vi "Get Tube Position Arrays.vi"(10 "PPR":i32=1024, 11 "Position Array":T2[](array[typedef])=[{"Positions"=enum."Tube Red A", "Count"=47}, {"Positions"=enum."Tube Black F", "Count"=213}, {"Positions"=enum."Tube Red E", "Count"=383}, {"Positions"=enum."Tube Black D", "Count"=557}, {"Positions"=enum."Tube Red C", "Count"=724}, {"Positions"=enum."Tube Black B", "Count"=898}]) -> (2 "Counts":i32[](array[numeric]), 3 "Positons":T1[](array[typedef]))   [LabVIEW 2020, in "Tube Wheel_ACT.lvlib"]
uses:
  Tube Wheel_ACT.lvlib
  Type Defs/Cluster_Tube Wheel Positions.ctl
  Shared Code/TypeDefs/ENUM_Tube Wheel Positions.ctl
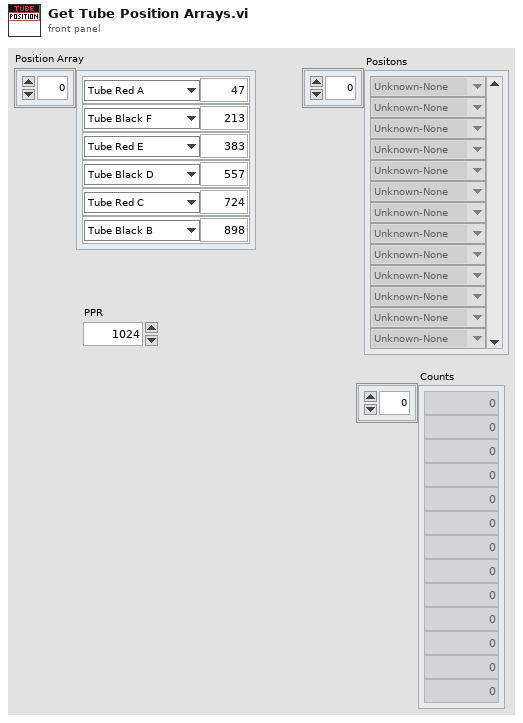
[diagram p1: front panel]
types:
  T1 = typedef "ENUM_Tube Wheel Positions.ctl" = enum16{"Unknown-None", "Tube Red A", "Tube Black B", "Tube Red C", "Tube Black D", "Tube Red E", "Tube Black F", "Load A-B", "Load B-C", "Load C-D", "Load D-E", "Load E-F", "Load F-A"}
  T2 = typedef "Cluster_Tube Wheel Positions.ctl" = cluster{"Positions":T1, "Count":i32}
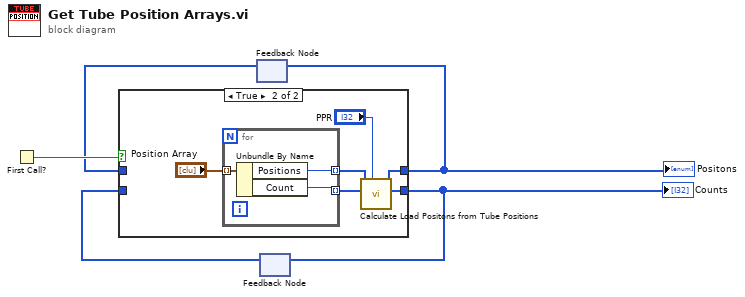
[diagram p0: block diagram]
diagram:
  n1 = First Call?() -> (First Call?: T/F=w5:bool)
  n2 = feedback #1() -> (w2:T1[])  [unwired: 1 in]
  n3 = feedback #2() -> (w1:i32[])  [unwired: 1 in]
  n4 = case shown="True" w5 {
    tunnel: [w7 w11] -> w4
    tunnel: [w6 w9] -> w3
    tunnel: w2 -> [w7 _]
    tunnel: w1 -> [w6 _]
    frame False {
    }
    frame True {
      n5 = for {
        tunnel: "Position Array" -> [w16] mode=indexing
        tunnel: [w15] -> w12 mode=indexing
        tunnel: [w14] -> w10 mode=indexing
        n6 = Unbundle By Name(w16) -> ("Positions"=w15:T1, "Count"=w14:i32)
      }
      n7 = call "Calculate Load Positons from Tube Positions.vi"("PPR"="PPR", "Tube Counts"=w10, "Tube Positions"=w12) -> ("Tube Counts Out"=w9:i32[], "Tube Positions Out"=w11:T1[])  [unwired: 7 in]
    }
  }
  "Counts" <- w3
  "Positons" <- w4
  n8 = feedback-in #1(w4) -> ()
  n9 = feedback-in #2(w3) -> ()
